vi "Initialise.vi"(6 "timeout in ms (-1)":i32=-1, 8 "error in (no error)":errorcluster, 11 "JQMHModule in":refnum<class "RQMHModule.lvclass">) -> (0 "error out":errorcluster, 1 "timed out?":bool, 2 "Did Init?":bool, 3 "JQMHModule out":refnum<class "RQMHModule.lvclass">)   [LabVIEW 2024, in "RQMHModule.lvclass"]
uses:
  RQMHModule.lvclass
  Reply.ctl
  InitialiseArgs.ctl
  RQMHModule.lvclass/RQMHModule.ctl
  InitialiseReplyArgs.ctl
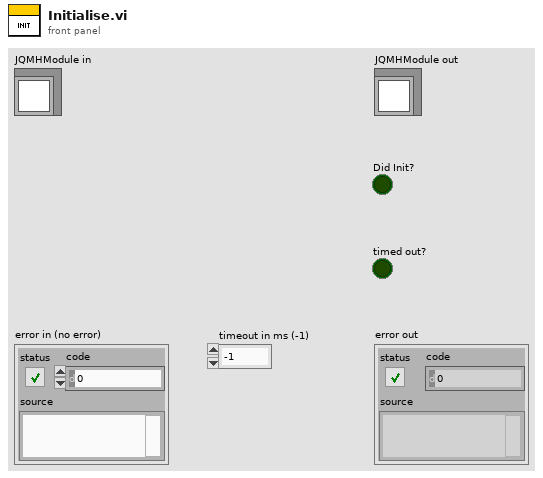
[diagram p1: front panel]
types:
  T1 = typedef "RQMHModule.lvclass/InitialiseArgs.ctl" = cluster{"null":bool}
  T2 = typedef "RQMHModule.lvclass/Reply.ctl" = cluster{"Expects Reply":bool, "Reply":refnum<notifier>}
  T3 = typedef "RQMHModule.lvclass/InitialiseReplyArgs.ctl" = cluster{"Did Init?":bool}
  T4 = cluster{"RQMH_REPLYARGS":T3, "error in (no error)":errorcluster}
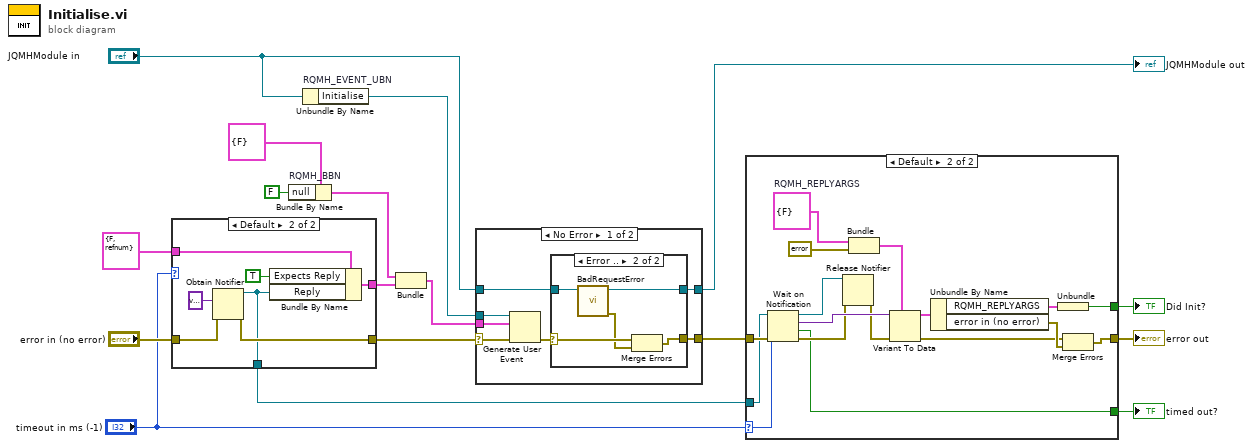
[diagram p0: block diagram]
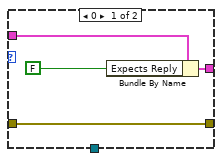
[diagram p4: hidden frame]
diagram:
  n1 = case shown="Default" "timeout in ms (-1)" {
    tunnel: [w20 w27] -> w13
    tunnel: "error in (no error)" -> [w18 w26]
    tunnel: [w18 w25] -> w10
    tunnel: [_ w24] -> w8
    tunnel: T2 {"Expects Reply"=FALSE, "Reply"=refnum} ("Reply") -> [w21 w23]
    frame 0 {
      n2 = Bundle By Name(cluster=w21, "Expects Reply"=FALSE) -> (w20:T2)
    }
    frame Default {
      n3 = Obtain Notifier(notification data type=variant, error in (no error)=w26) -> (notifier out=w24:refnum<notifier>, error out=w25:errorcluster)  [unwired: 2 in, 1 out]
      n4 = Bundle By Name(cluster=w23, "Expects Reply"=TRUE, "Reply"=w24) -> (w27:T2)
    }
  }
  n5 = Bundle By Name "RQMH_BBN"(cluster=T1 {"null"=FALSE} ("Args"), "null"=FALSE) -> (w14:T1)
  n6 = Unbundle By Name "RQMH_EVENT_UBN"("JQMHModule in") -> ("Initialise"=w17:refnum<user-event>)
  n7 = Bundle("Args"=w14, "Reply"=w13) -> (w12:cluster{"Args":T1, "Reply":T2})  [unwired: 1 in]
  n8 = case shown="No Error" w10 {
    selector: w10 -> [w32 w43]
    tunnel: w12 -> [w35 _]
    tunnel: w17 -> [w34 _]
    tunnel: [w31 w43] -> w9
    tunnel: "JQMHModule in" -> [w30 w44]
    tunnel: [w29 w44] -> w15
    frame No Error {
      n9 = Generate User Event(user event=w34, event data cluster=w35, error in=w32) -> (error out=w33:errorcluster)  [unwired: 1 in, 1 out]
      n10 = case shown="Error .." w33 {
        selector: w33 -> [w36 w42]
        tunnel: [w36 w41] -> w31
        tunnel: w30 -> [w37 w40]
        tunnel: [w37 w39] -> w29
        frame No Error {
        }
        frame Error {
          n11 = call "BadRequestError.vi"("JQMHModule in"=w40) -> ("error out"=w38:errorcluster, "JQMHModule out"=w39:refnum<class "RQMHModule.lvclass">)  [unwired: 9 in]
          n12 = Merge Errors(w42, w38) -> (w41:errorcluster)
        }
      }
    }
    frame Error {
    }
  }
  "JQMHModule out" <- w15
  n13 = case shown="Default" "timeout in ms (-1)" {
    selector: "timeout in ms (-1)" -> [_ w48]
    tunnel: w9 -> [w45 w62]
    tunnel: w8 -> [_ w61]
    tunnel: [w45 w54] -> w7
    tunnel: [_ w50] -> w6
    tunnel: [_ w46] -> w1
    frame 0 {
    }
    frame Default {
      w47 = T3 {"Did Init?"=FALSE}  # RQMH_REPLYARGS
      n14 = Wait on Notification(notifier=w61, timeout in ms (-1)=w48, error in (no error)=w62) -> (notifier out=w53:refnum<notifier>, notification=w58:variant, timed out?=w50:bool, error out=w52:errorcluster)  [unwired: 1 in]
      n15 = Release Notifier(notifier=w53, error in (no error)=w52) -> (error out=w51:errorcluster)  [unwired: 1 in, 2 out]
      n16 = Bundle("RQMH_REPLYARGS"=w47, "error in (no error)"=errorcluster {"status"=FALSE, "code"=0, "source"=""}) -> (w60:T4)  [unwired: 1 in]
      n17 = Variant To Data(error in=w51, type=w60, Variant=w58) -> (data=w57:T4, error out=w55:errorcluster)
      n18 = Unbundle By Name(w57) -> ("RQMH_REPLYARGS"=w49:T3, "error in (no error)"=w56:errorcluster)
      n19 = Unbundle(w49) -> ("Did Init?"=w46:bool)
      n20 = Merge Errors(w55, w56) -> (w54:errorcluster)
    }
  }
  "error out" <- w7
  "timed out?" <- w6
  "Did Init?" <- w1
